vi "close.vi"(8 "error in (no error)":errorcluster caption="错误输入（无错误）", 11 "Primary Productivity 输入":refnum<class "Primary Productivity.lvclass">) -> (0 "error out":errorcluster caption="错误输出", 3 "Primary Productivity 输出":refnum<class "Primary Productivity.lvclass">)   [LabVIEW 2016, in "Primary Productivity.lvclass"]
uses:
  Primary Productivity.lvclass
  Primary Productivity.lvclass/Primary Productivity.ctl
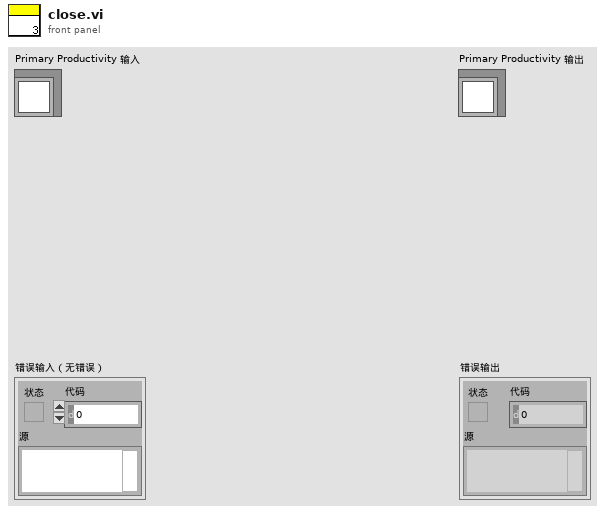
[diagram p1: front panel]
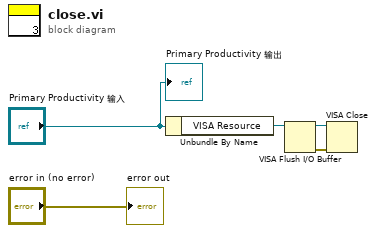
[diagram p0: block diagram]
diagram:
  n1 = Unbundle By Name("Primary Productivity 输入") -> ("VISA Resource"=w3:refnum<visa-resource-name>)
  n2 = VISA Flush I/O Buffer(VISA resource name=w3) -> (VISA resource name out=w2:refnum<visa-resource-name>, error out=w1:errorcluster)  [unwired: 2 in]
  n3 = VISA Close(VISA resource name=w2, error in (no error)=w1) -> ()  [unwired: 1 out]
  "error out" <- "error in (no error)"
  "Primary Productivity 输出" <- "Primary Productivity 输入"
